vi "Load Index from File.vi"(8 "error in (no error)":errorcluster, 10 "Project or Class Path":path, 11 "Bufferend Test Finder in":refnum<class "Indexing Test Finder.lvclass">) -> (0 "error out":errorcluster, 3 "Bufferend Test Finder out":refnum<class "Indexing Test Finder.lvclass">)   [LabVIEW 2020, in "Indexing Test Finder.lvclass"]
uses:
  Indexing Test Finder.lvclass
  Indexing Test Finder.lvclass/Indexing Test Finder.ctl
  TypeDefs/Index Item.ctl
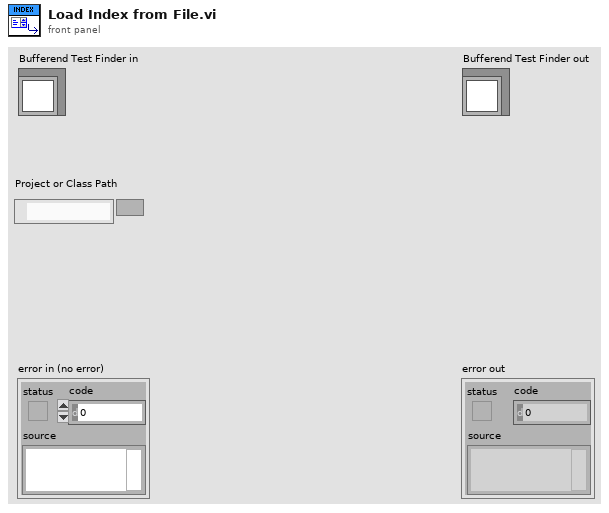
[diagram p1: front panel]
types:
  T1 = enum16{"open", "replace", "create", "open or create", "replace or create", "replace or create with confirmation"}
  T2 = typedef "Indexing Test Finder.lvclass/Index Item.ctl" = cluster{"Dynamic Methods":map{string, path}, "Static Methods":map{string, path}, "Signature":string}
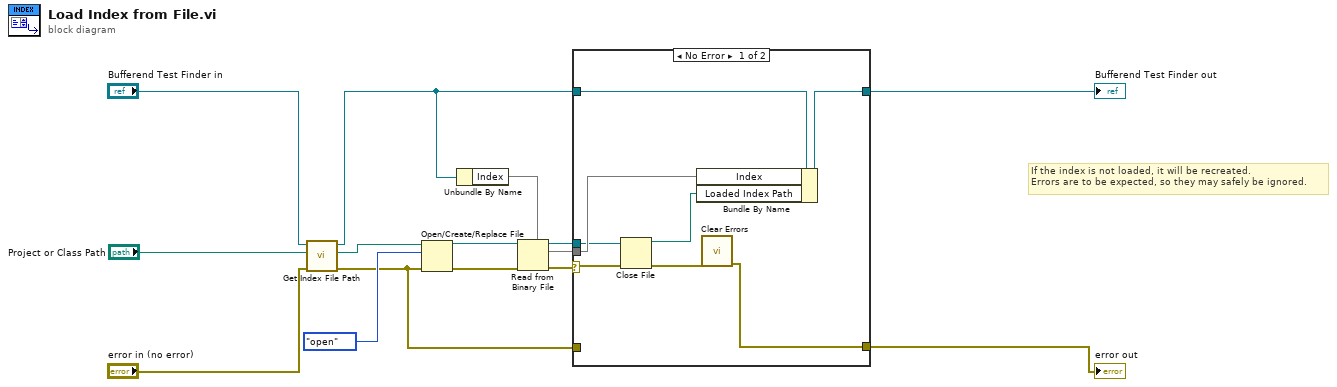
[diagram p0: block diagram]
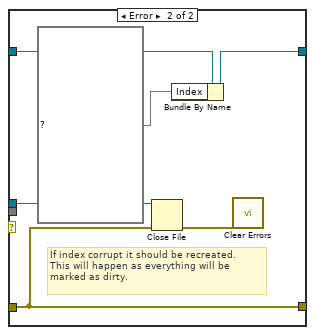
[diagram p2: hidden frame]
diagram:
  # "If the index is not loaded, it will be recreated.\nErrors are to be expected, so they may safely be ignored."
  n1 = call "Get Index File Path.vi"("error in (no error)"="error in (no error)", "Project or Class Path"="Project or Class Path", "Indexing Test Finder in"="Bufferend Test Finder in") -> ("error out"=w5:errorcluster, "Index File Path"=w2:path, "Indexing Test Finder out"=w6:refnum<class "Indexing Test Finder.lvclass">)  [unwired: 6 in]
  n2 = Open/Create/Replace File(file path (use dialog)=w2, error in=w5, operation (0:open)=T1."open") -> (refnum out=w13:refnum<file>, error out=w12:errorcluster)  [unwired: 3 in, 1 out]
  n3 = Unbundle By Name(w6) -> ("Index"=w11:map{path, T2})
  n4 = Read from Binary File(5:w11, 8:w12, 11:w13) -> (0:w9:errorcluster, 2:w10:map{path, T2}, 3:w8:refnum<file>)  [unwired: 3 in, 1 out]
  n5 = case shown="No Error" w9 {
    selector: w9 -> [w16 _]
    tunnel: [w23 w28] -> w15
    tunnel: w6 -> [w22 w29]
    tunnel: w10 -> [w21 _]
    tunnel: w8 -> [w20 w25]
    tunnel: w5 -> [_ w24]
    tunnel: [w19 w24] -> w1
    frame No Error {
      n6 = Close File(refnum=w20, error in=w16) -> (path=w17:path, error out=w18:errorcluster)
      n7 = Bundle By Name(cluster=w22, "Index"=w21, "Loaded Index Path"=w17) -> (w23:refnum<class "Indexing Test Finder.lvclass">)
      n8 = call <vilib>:"Clear Errors.vi"("error in (no error)"=w18) -> ("error out"=w19:errorcluster)  [unwired: 5 in, 1 out]
    }
    frame Error {
      # "If index corrupt it should be recreated.\nThis will happen as everything will be marked as dirty."
      n9 = Close File(refnum=w25, error in=w24) -> (error out=w26:errorcluster)  [unwired: 1 out]
      n10 = Bundle By Name(cluster=w29, "Index"=map{path, T2} {}) -> (w28:refnum<class "Indexing Test Finder.lvclass">)
      n11 = call <vilib>:"Clear Errors.vi"("error in (no error)"=w26) -> ()  [unwired: 5 in, 2 out]
    }
  }
  "error out" <- w1
  "Bufferend Test Finder out" <- w15
